vi "Write Current Edit Position.vi"(8 "error in (no error)":errorcluster, 10 "Current Edit Position":T1, 11 "DataGrid in":refnum<class "DataGrid.lvclass">) -> (0 "error out":errorcluster, 3 "DataGrid out":refnum<class "DataGrid.lvclass">)   [LabVIEW 2017, in "DataGrid.lvclass"]
uses:
  DataGrid.lvclass
  <vilib>/Utility/miscctls.llb/LVRowAndColumnTypeDef.ctl
  DataGrid.lvclass/DataGrid.ctl
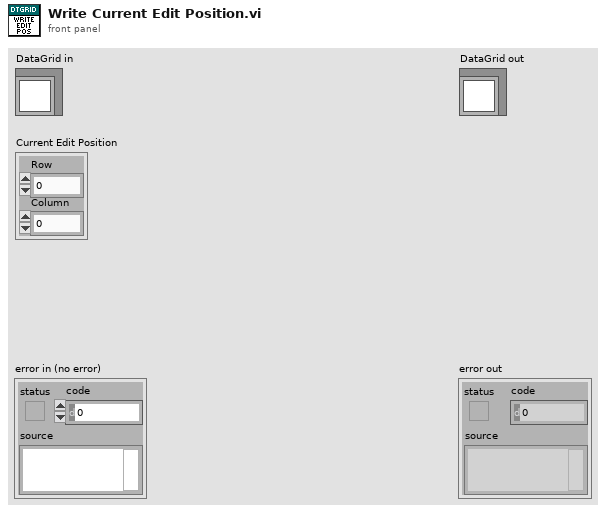
[diagram p1: front panel]
types:
  T1 = typedef "LVRowAndColumnTypeDef.ctl" = cluster{"Row":i32, "Column":i32}
  T2 = typedef "DataGrid.lvclass/State Data.ctl" = cluster{"Config":refnum<class "DataGrid Config.lvclass">, "Current Edit Position":T1}
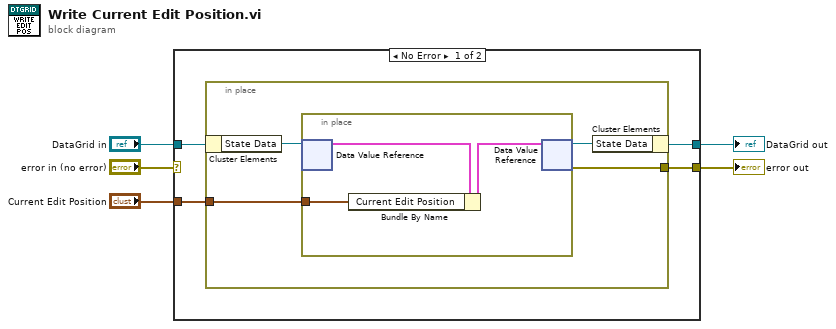
[diagram p0: block diagram]
diagram:
  n1 = case shown="No Error" "error in (no error)" {
    selector: "error in (no error)" -> [_ w18]
    tunnel: [w6 w18] -> w4
    tunnel: [w7 w17] -> w2
    tunnel: "DataGrid in" -> [w9 w17]
    tunnel: "Current Edit Position" -> [w8 _]
    frame No Error {
      n2 = in-place {
        in-place-border: w8 -> [w12]
        in-place-border: [w10] -> w6
        n3 = in-place-cluster #1(w9) -> ("State Data"=w13:refnum<data-value>)
        n4 = in-place {
          in-place-border: w12 -> [w15]
          n5 = in-place-dvr #2(w13) -> (w16:T2)  [unwired: 1 out]
          n6 = Bundle By Name(cluster=w16, "Current Edit Position"=w15) -> (w14:T2)
          n7 = in-place-dvr #2(w14) -> (w11:refnum<data-value>, w10:errorcluster)
        }
        n8 = in-place-cluster #1("State Data"=w11) -> (w7:refnum<class "DataGrid.lvclass">)
      }
    }
    frame Error {
    }
  }
  "error out" <- w4
  "DataGrid out" <- w2
